vi "Tank.vi"() -> ()   [LabVIEW 2016]
panel:
  out "Tank":dbl(slide) scale=0.0..1.0
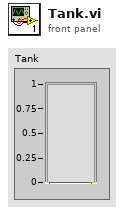
[diagram p1: front panel]
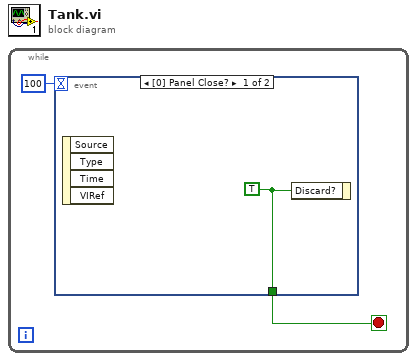
[diagram p0: block diagram]
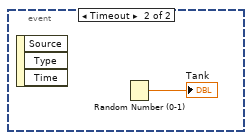
[diagram p2: hidden frame]
diagram:
  n1 = while {
    stop <- w1 stop-if-true
    n2 = event shown="[0] Panel Close?" {
      selector: _ -> [_ _]
      dyn-events: _ -> [_ _]
      timeout: 100 -> [_ _]
      tunnel: [w3 _] -> w1
      event Panel Close? {
        w3 = TRUE ("Discard?")
        n3 = event-data() -> ()  [unwired: 1 in, 4 out]
        n4 = event-data("Discard?"=w3) -> ()  [unwired: 1 in, 1 out]
      }
      event Timeout {
        n5 = event-data() -> ()  [unwired: 1 in, 3 out]
        n6 = Random Number (0-1)() -> (number: 0 to 1=→"Tank":dbl)
      }
    }
  }
